vi "Dashboard Main.vi"() -> ()   [LabVIEW 2012]
uses:
  <vilib>/event_ctls.llb/eventvkey.ctl
  <vilib>/Utility/config.llb/Read Key (String).vi
  <vilib>/Utility/config.llb/Read Key (I32).vi
  <vilib>/Utility/config.llb/Write Key (String).vi
  <vilib>/Utility/config.llb/Write Key (I32).vi
  <vilib>/Utility/config.llb/NI_LVConfig.lvlib
panel:
  out "Mode":T1(ring)=enum."Auto Disabled"
  in  "Viewer":enum32{"Camera Image", "Variables"}(tab)
  out "Mbps":dbl format="%#.1g"
  in  "Enable":bool=TRUE
  in  "DB Camera Config":bool
  out "Mbps":bool
  out "fps":dbl format="%#.1g"
  out "Image Error Message":string="Timeout in Camera Communications"
  out "Camera Image":T2(plugin-control)
  out "Camera Image 2":T2(plugin-control)
  in  "Camera Settings":T3={"Frame Rate"=15, "Compression"=30, "Size"=1} {"Frame Rate" scale=1.0..30.0; "Size" items=["640x480", "320x240", "160x120"]}
  out "Camera IP 2":string
  out "Camera IP":string
  out "fps 2":dbl format="%#.1g"
  out "Mbps 2":dbl format="%#.1g"
  in  "Enable 2":bool=TRUE
  in  "FR":i32=15
  out "Tree":string(tree)
  in  "Dashboard Tab":enum32{"Operation", "Test", "Checklist"}(tab)
  in  "Auton Selector":T4(radio)
  in  "Auton Refresh":bool
  out "AutonFiles":string[](array[string])
  in  "Slider":dbl(slide) scale=0.0..100.0 scale format="%#_3g"
  in  "On/Off":bool caption="Solenoid"
  in  "Test Name":u16(ring) items=["Select the test to run...", "Example Test", "-------------------------------", "List of tests is built in robot code.", "Replace with your own automated tests."]
  in  "Test Tree":string(tree)
  in  "Motor":cluster{"Value":dbl, "Enable":bool} {"Value" scale=-1.0..1.0 scale format="%#_3g"}
  out "Progress":T5 {"Test Progress" scale=0.0..100.0}
  in  "Rev/Fwd":cluster{"Forward":bool, "Reverse":bool}
  in  "Ring":u16(ring) items=["Auto", "Fixed indoor", "Fixed outdoor 1", "Fixed outdoor 2", "Fixed fluorescent 1", "Fixed fluorescent 2", "Hold current"]
  in  "Listbox":i32(listbox)
  out "Robot IP":string
  out "Battery Value":dbl(slide) scale=0.0..14.0 scale format="%#_2e"
  out "Battery":sgl(graph)
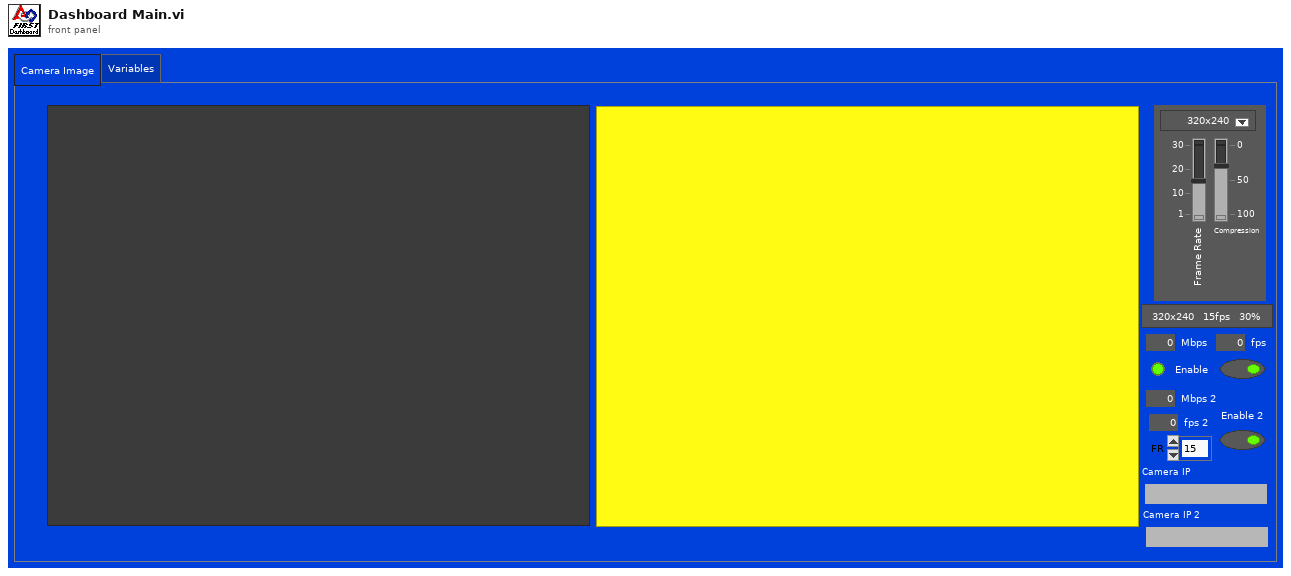
[diagram p1: front panel]
types:
  T1 = enum8{"Tele-Op Disabled", "Tele-Op Enabled", "Auto Disabled", "Auto Enabled", "Test Disabled", "Test Enabled", ""}
  T2 = typedef "IMAQ Image.ctl" = refnum<image>
  T3 = cluster{"Frame Rate":i32, "Compression":i32, "Size":u16}
  T4 = enum32{"Boolean 1", "Boolean 2", "Boolean 3", "Boolean 4", "Boolean 5", "Boolean 6", "Boolean 7", "Boolean 8"}
  T5 = cluster{"Test Progress":u8, "Test Progress Text":string}
  T6 = typedef "Image Type" = u32
  T7 = cluster{"Competition mode":bool, "Robot Link":bool, "Autonomous":bool, "Enabled":bool, "E-Stop":bool, "Simulated":bool, "TestMode":bool, "Docked Window":bool}
  T8 = typedef "LVRectTypeDef.ctl" = cluster{"Left":i16, "Top":i16, "Right":i16, "Bottom":i16}
  T9 = typedef "NI_LVConfig.lvlib/Config Data RefNum.ctl" = refnum<k1>
  T10 = typedef "eventvkey.ctl" = enum16{"ASCII", "Enter", "Return", "Shift", "Ctrl", "Alt", "Cmd", "Opt", "Caps", "NumLock", "Clear", "Break", "Up", "Down", "Left", "Right", "Insert", "Delete", "Home", "End", "PageUp", "PageDown", "Escape", "Help", "Pause", "ScrollLock", "F1", "F2", "F3", "F4", "F5", "F6", "F7", "F8", "F9", "F10", "F11", "F12", "F13", "F14", "F15", "F16", "F17", "F18", "F19", "F20", "F21", "F22", "F23", "F24", "Play", "VolumeUp", "VolumeDown", "Mute", "Two Byte Char"}
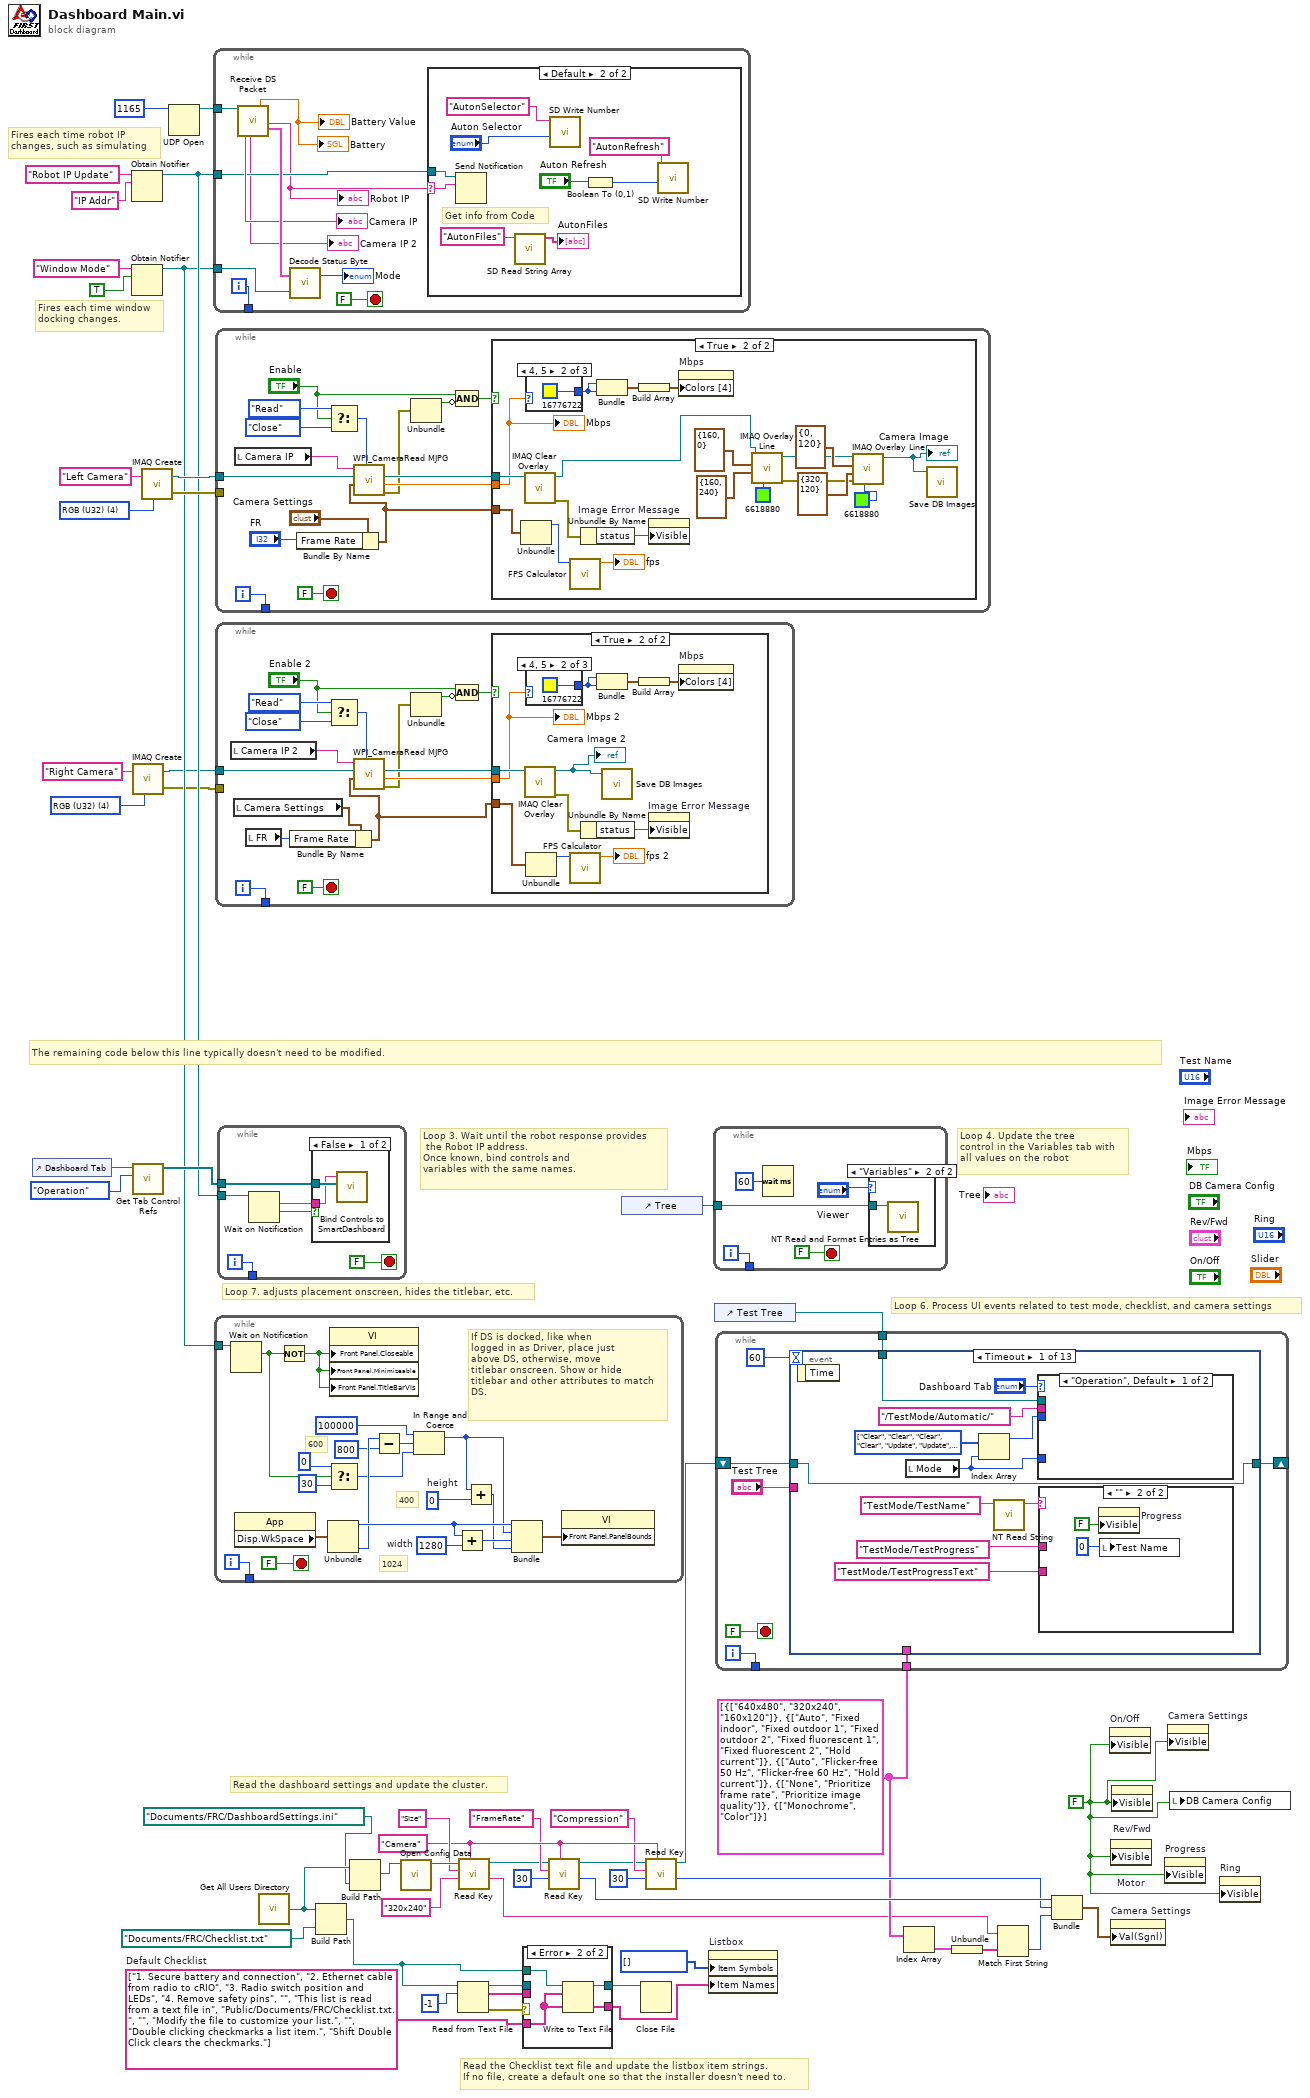
[diagram p0: block diagram]
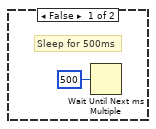
[diagram p2: hidden frame]
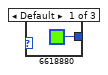
[diagram p3: hidden frame]
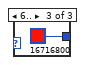
[diagram p4: hidden frame]
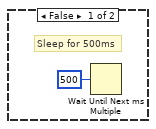
[diagram p6: hidden frame]
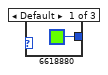
[diagram p7: hidden frame]
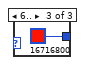
[diagram p8: hidden frame]
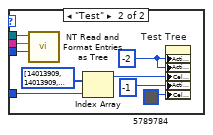
[diagram p10: hidden frame]
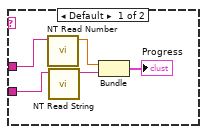
[diagram p11: hidden frame]
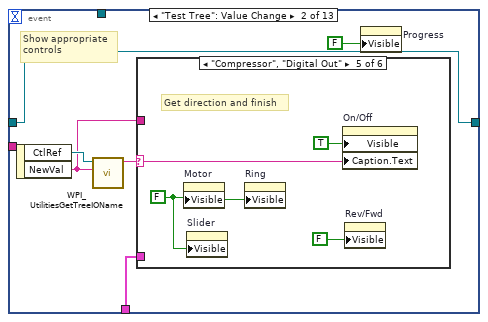
[diagram p12: hidden frame]
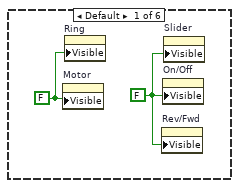
[diagram p13: hidden frame]
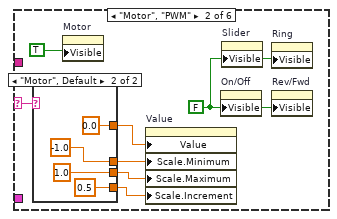
[diagram p14: hidden frame]
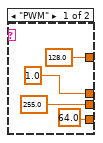
[diagram p15: hidden frame]
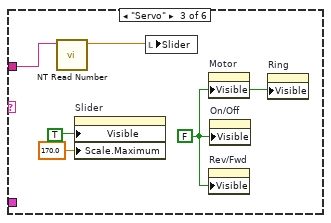
[diagram p16: hidden frame]
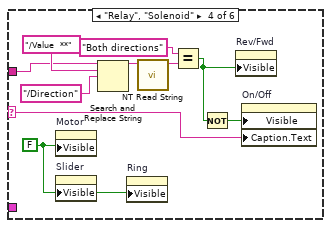
[diagram p17: hidden frame]
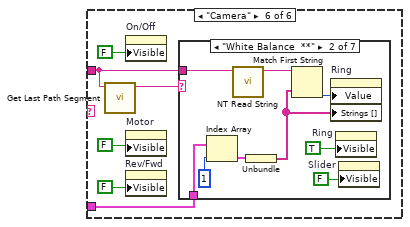
[diagram p18: hidden frame]
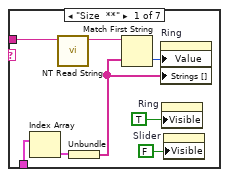
[diagram p19: hidden frame]
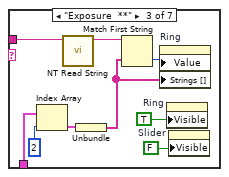
[diagram p20: hidden frame]
diagram:
  w3 = T6 4 items=["Grayscale (U8)", "Grayscale (I16)", "Grayscale (SGL)", "Complex (CSG)", "RGB (U32)", "HSL (U32)", "RGB (U64)"] ("Image Type")
  w25 = "Camera"
  w17 = cluster{string[]}[] [{["640x480", "320x240", "160x120"]}, {["Auto", "Fixed indoor", "Fixed outdoor 1", "Fixed outdoor 2", "Fixed fluorescent 1", "Fixed fluorescent 2", "Hold current"]}, {["Auto", "Flicker-free 50 Hz", "Flicker-free 60 Hz", "Hold current"]}, {["None", "Prioritize frame rate", "Prioritize image quality"]}, {["Monochrome", "Color"]}]
  w33 = string[] ["1. Secure battery and connection", "2. Ethernet cable from radio to cRIO", "3. Radio switch position and LEDs", "4. Remove safety pins", "", "This list is read from a text file in", "Public/Documents/FRC/Checklist.txt.", "", "Modify the file to customize your list.", "", "Double clicking checkmarks a list item.", "Shift Double Click clears the checkmarks."]  # Default Checklist
  w31 = FALSE ("Visible")
  w52 = T6 4 items=["Grayscale (U8)", "Grayscale (I16)", "Grayscale (SGL)", "Complex (CSG)", "RGB (U32)", "HSL (U32)", "RGB (U64)"] ("Image Type")
  # "Fires each time robot IP\nchanges, such as simulating"
  # "Fires each time window\ndocking changes."
  # "Read the Checklist text file and update the listbox item strings.\nIf no file, create a default one so that the installer doesn't need to."
  # "The remaining code below this line typically doesn't need to be modified."
  # "Loop 6. Process UI events related to test mode, checklist, and camera settings"
  # "Read the dashboard settings and update the cluster."
  # "Loop 4. Update the tree\ncontrol in the Variables tab with\nall values on the robot"
  # "Loop 3. Wait until the robot response provides\n the Robot IP address.\nOnce known, bind controls and\nvariables with the same names."
  # "Loop 7. adjusts placement onscreen, hides the titlebar, etc."
  n1 = control-ref of="Dashboard Tab"() -> (w47:refnum<vi>)
  n2 = Obtain Notifier(name (unnamed)="Robot IP Update", notification data type="IP Addr" ("name (unnamed)")) -> (notifier out=w44:refnum<notifier>)  [unwired: 2 in, 2 out]
  n3 = Obtain Notifier(name (unnamed)="Window Mode", notification data type=TRUE) -> (notifier out=w37:refnum<notifier>)  [unwired: 2 in, 2 out]
  n4 = call "IMAQ Create"("Image Name"="Right Camera", "Image Type"=w3) -> ("New Image"=w2:T2, "error out"=w1:errorcluster)  [unwired: 2 in, 1 out]
  n5 = call <vilib>:"Get Tab Control Refs.vi"("Page Index"=enum32{"Operation", "Test"}."Operation" ("Dashboard Tab"), "TabControl in"=w47) -> ("ControlsOnPage"=w48:refnum<vi>[])  [unwired: 9 in]
  n6 = call "IMAQ Create"("Image Name"="Left Camera", "Image Type"=w52) -> ("New Image"=w50:T2, "error out"=w49:errorcluster)  [unwired: 2 in, 1 out]
  n7 = UDP Open(11:u16 1165 ("port")) -> (port=w53:refnum<k16>)  [unwired: 2 in, 4 out]
  n8 = while {
    tunnel: w53 -> [w63]
    tunnel: w44 -> [w57]
    tunnel: w37 -> [w61]
    tunnel: [w58] -> _
    i -> [w58]
    stop <- FALSE stop-if-true
    n9 = call "Receive DS Packet.vi"("Recv Socket"=w63) -> ("Camera IP Address"=→"Camera IP":string, "Camera IP Address 2"=→"Camera IP 2":string, "Battery"=→"Battery" →"Battery Value":sgl, "Robot IP Address"=w56:string, "Status"=w64:T7)  [unwired: 8 in, 6 out]
    "Robot IP" <- w56
    n10 = call "Decode Status Byte.vi"("Window Mode Notifier"=w61, "Status"=w64) -> ("Mode"=→"Mode":T1)  [unwired: 1 out]
    n11 = case shown="Default" w56 {
      selector: w56 -> [_ w73]
      tunnel: w57 -> [_ w74]
      frame "0.0.0.0" {
        # "Robot not responding, don't poll the variables"
      }
      frame Default {
        # "Get info from Code"
        n12 = Send Notification(notification=w73, notifier=w74) -> ()  [unwired: 1 in, 2 out]
        n13 = call <vilib>:"SD Read String Array.vi"("Name"="AutonFiles") -> ("String Array"=→"AutonFiles":string[])  [unwired: 9 in, 1 out]
        n14 = call <vilib>:"SD Write Number.vi"("Numeric"="Auton Selector", "Name"="AutonSelector") -> ()  [unwired: 8 in, 2 out]
        n15 = Boolean To (0,1)(Boolean="Auton Refresh") -> (0, 1=w67:i16)
        n16 = call <vilib>:"SD Write Number.vi"("Numeric"=w67, "Name"="AutonRefresh") -> ()  [unwired: 8 in, 2 out]
      }
    }
  }
  n17 = while {
    tunnel: w37 -> [w93]
    tunnel: [w91] -> _
    i -> [w91]
    stop <- FALSE stop-if-true
    w83 = 1280  # width
    w86 = 0  # height
    # "600"
    # "1024"
    # "400"
    # "If DS is docked, like when\nlogged in as Driver, place just\nabove DS, otherwise, move\ntitlebar onscreen. Show or hide\ntitlebar and other attributes to match\nDS."
    n18 = Wait on Notification(notifier=w93) -> (notification=w78:bool)  [unwired: 3 in, 3 out]
    n19 = property class="App"() -> ("Disp.WkSpace"=w89:T8)  [unwired: 2 in, 2 out]
    n20 = Not(x=w78) -> (.not. x?=w92:bool)
    n21 = Unbundle(w89) -> ("Left"=w87:i16, "Bottom"=w84:i16)  [unwired: 2 out]
    n22 = Select(t=0, s=w78, f=30) -> (s? t:f=w77:i32)
    n23 = property class="VI"("Front Panel.Closeable"=w92, "Front Panel.Minimizeable"=w92, "Front Panel.TitleBarVis"=w92) -> ()  [unwired: 2 in, 2 out]
    n24 = Subtract(x=w84, y=800) -> (x-y=w81:i32)
    n25 = In Range and Coerce(upper limit=100000, x=w81, lower limit=w77) -> (coerced(x)=w75:i32)  [unwired: 1 out]
    n26 = Add(x=w87, y=w83) -> (x+y=w88:i32)
    n27 = Add(x=w75, y=w86) -> (x+y=w85:i32)
    n28 = Bundle("Left"=w87, w75, w88, w85) -> (w90:cluster{"Left":i16, i32, i32, i32})  [unwired: 1 out]
    n29 = property class="VI"("Front Panel.PanelBounds"=w90) -> ()  [unwired: 2 in, 2 out]
  }
  n30 = while {
    tunnel: w50 -> [w107]
    tunnel: w49 -> [_]
    tunnel: [w109] -> _
    i -> [w109]
    stop <- FALSE stop-if-true
    n31 = local read "Camera IP"() -> (w108:string)
    n32 = Bundle By Name(cluster="Camera Settings", "Frame Rate"="FR") -> (w95:T3)
    n33 = Select(t=enum16{"Read", "Reopen", "Close"}."Read" ("Operation"), s="Enable", f=enum16{"Read", "Reopen", "Close"}."Close" ("Operation")) -> (s? t:f=w102:enum16{"Read", "Reopen", "Close"})
    n34 = call <vilib>:"WPI_CameraRead MJPG.vi"("Operation"=w102, "Camera Settings"=w95, "Image"=w107, "address"=w108) -> ("error out"=w101:errorcluster, "Bandwidth (kbps)"=w105:dbl, "Image Out"=w106:T2)  [unwired: 5 in]
    n35 = Unbundle(w101) -> ("status"=w99:bool)  [unwired: 2 out]
    n36 = Compound Arithmetic op=AND("Enable", invert w99) -> (w98:bool)
    n37 = case shown="True" w98 {
      tunnel: w95 -> [_ w123]
      tunnel: w106 -> [_ w126]
      tunnel: w105 -> [_ w125]
      frame False {
        # "Sleep for 500ms"
        n38 = Wait Until Next ms Multiple(millisecond multiple=u32 500) -> ()  [unwired: 1 out]
      }
      frame True {
        n39 = Unbundle(w123) -> ("Frame Rate"=w113:i32)  [unwired: 2 out]
        n40 = call "IMAQ Clear Overlay"("Image"=w126) -> ("error out"=w130:errorcluster, "Image Out"=w115:T2)  [unwired: 2 in, 7 out]
        n41 = case shown="4, 5" w125 {
          tunnel: [u32 6618880 ("Color Box") u32 16776722 ("Color Box") u32 16716800 ("Color Box")] -> w127
          frame Default {
          }
          frame 4, 5 {
          }
          frame 6.. {
          }
        }
        n42 = call "FPS Calculator.vi"("Average Count"=w113) -> ("fps"=→"fps":dbl)  [unwired: 10 in]
        n43 = Unbundle By Name(w130) -> ("status"=w131:bool)
        n44 = Bundle("Color Box"=w127, "Color Box"=w127) -> (w129:cluster{"Color Box":u32, "Color Box":u32})  [unwired: 1 out]
        n45 = Build Array(w129) -> (w128:cluster{"Color Box":u32, "Color Box":u32}[])
        n46 = property on="Image Error Message" class="Str"("Visible"=w131) -> ()  [unwired: 2 in, 2 out]
        n47 = property on="Mbps" class="Bool (strict)"("Colors [4]"=w128) -> ()  [unwired: 2 in, 2 out]
        n48 = call "IMAQ Overlay Line"("Color"=u32 6618880, "End Point"=cluster{"X":i32, "Y":i32} {"X"=160, "Y"=240}, "Start Point"=cluster{"X":i32, "Y":i32} {"X"=160, "Y"=0}, "Image"=w115) -> ("error out"=w120:errorcluster, "Image Out"=w119:T2)  [unwired: 6 in]
        n49 = call "IMAQ Overlay Line"("Color"=u32 6618880, "error in (no error)"=w120, "End Point"=cluster{"X":i32, "Y":i32} {"X"=320, "Y"=120}, "Start Point"=cluster{"X":i32, "Y":i32} {"X"=0, "Y"=120}, "Image"=w119) -> ("Image Out"=w114:T2)  [unwired: 5 in, 1 out]
        "Camera Image" <- w114
        n50 = call "Save DB Images.vi"("Image"=w114) -> ()  [unwired: 2 in, 1 out]
        "Mbps" <- w125
      }
    }
  }
  n51 = while {
    tunnel: w2 -> [w147]
    tunnel: [w149] -> _
    tunnel: w1 -> [_]
    i -> [w149]
    stop <- FALSE stop-if-true
    n52 = local read "Camera IP 2"() -> (w148:string)
    n53 = local read "Camera Settings"() -> (w136:T3)
    n54 = local read "FR"() -> (w137:i32)
    n55 = Bundle By Name(cluster=w136, "Frame Rate"=w137) -> (w135:T3)
    n56 = Select(t=enum16{"Read", "Reopen", "Close"}."Read" ("Operation"), s="Enable 2", f=enum16{"Read", "Reopen", "Close"}."Close" ("Operation")) -> (s? t:f=w142:enum16{"Read", "Reopen", "Close"})
    n57 = call <vilib>:"WPI_CameraRead MJPG.vi"("Operation"=w142, "Camera Settings"=w135, "Image"=w147, "address"=w148) -> ("error out"=w141:errorcluster, "Bandwidth (kbps)"=w145:dbl, "Image Out"=w146:T2)  [unwired: 5 in]
    n58 = Unbundle(w141) -> ("status"=w139:bool)  [unwired: 2 out]
    n59 = Compound Arithmetic op=AND("Enable 2", invert w139) -> (w138:bool)
    n60 = case shown="True" w138 {
      tunnel: w135 -> [_ w154]
      tunnel: w146 -> [_ w157]
      tunnel: w145 -> [_ w156]
      frame False {
        # "Sleep for 500ms"
        n61 = Wait Until Next ms Multiple(millisecond multiple=u32 500) -> ()  [unwired: 1 out]
      }
      frame True {
        n62 = call "IMAQ Clear Overlay"("Image"=w157) -> ("error out"=w161:errorcluster, "Image Out"=w152:T2)  [unwired: 2 in, 7 out]
        "Camera Image 2" <- w152
        n63 = case shown="4, 5" w156 {
          tunnel: [u32 6618880 ("Color Box") u32 16776722 ("Color Box") u32 16716800 ("Color Box")] -> w158
          frame Default {
          }
          frame 4, 5 {
          }
          frame 6.. {
          }
        }
        n64 = Unbundle(w154) -> ("Frame Rate"=w153:i32)  [unwired: 2 out]
        n65 = call "FPS Calculator.vi"("Average Count"=w153) -> ("fps"=→"fps 2":dbl)  [unwired: 10 in]
        n66 = Unbundle By Name(w161) -> ("status"=w162:bool)
        n67 = Bundle("Color Box"=w158, "Color Box"=w158) -> (w160:cluster{"Color Box":u32, "Color Box":u32})  [unwired: 1 out]
        n68 = call "Save DB Images.vi"("Image"=w152) -> ()  [unwired: 2 in, 1 out]
        n69 = Build Array(w160) -> (w159:cluster{"Color Box":u32, "Color Box":u32}[])
        n70 = property on="Image Error Message" class="Str"("Visible"=w162) -> ()  [unwired: 2 in, 2 out]
        n71 = property on="Mbps" class="Bool (strict)"("Colors [4]"=w159) -> ()  [unwired: 2 in, 2 out]
        "Mbps 2" <- w156
      }
    }
  }
  n72 = while {
    tunnel: w48 -> [w171]
    tunnel: w44 -> [w168]
    tunnel: [w166] -> _
    i -> [w166]
    stop <- FALSE stop-if-true
    n73 = Wait on Notification(notifier=w168) -> (notification=w167:string, timed out?=w169:bool)  [unwired: 3 in, 2 out]
    n74 = case shown="False" w169 {
      tunnel: w171 -> [w173 _]
      tunnel: w167 -> [w172 _]
      frame False {
        n75 = call <vilib>:"Bind Controls to SmartDashboard.vi"("Bound Control Refs"=w173, "Server IP Address"=w172) -> ()  [unwired: 10 in]
      }
      frame True {
      }
    }
  }
  n76 = call "Get All Users Directory.vi"() -> ("All User Path"=w30:path)
  n77 = Build Path(base path=w30, name or relative path=path "Documents/FRC/Checklist.txt") -> (appended path=w34:path)
  n78 = Build Path(base path=w30, name or relative path=path "Documents/FRC/DashboardSettings.ini") -> (appended path=w29:path)
  n79 = call <vilib>:"Open Config Data.vi"("configuration file path"=w29) -> ("refnum"=w28:T9)  [unwired: 8 in, 2 out]
  n80 = Read from Text File(file (use dialog)=w34, count=-1 ("timeout ms (25000)")) -> (refnum out=w12:refnum<file>, text=w35:string[], error out=w36:errorcluster)  [unwired: 2 in, 1 out]
  n81 = call-poly <vilib>:"Read Key.vi"("section"=w25, "default value"="320x240", "key"="Size", "refnum"=w28) -> ("value"=w15:string, "refnum out"=w10:T9)  [unwired: 2 in, 4 out]
  n82 = case shown="Error" w36 {
    tunnel: w35 -> [w175 _]
    tunnel: [w175 w177] -> w32
    tunnel: w33 -> [_ w177]
    tunnel: w34 -> [_ w178]
    tunnel: [w174 w176] -> w11
    tunnel: w12 -> [w174 _]
    frame No Error {
    }
    frame Error {
      n83 = Write to Text File(file (use dialog)=w178, text=w177) -> (refnum out=w176:refnum<file>)  [unwired: 2 in, 2 out]
    }
  }
  n84 = call-poly <vilib>:"Read Key.vi"("section"=w25, "default value"=30, "key"="FrameRate", "refnum"=w10) -> ("value"=w20:i32, "refnum out"=w9:T9)  [unwired: 1 in, 5 out]
  n85 = control-ref of="Tree"() -> (w6:refnum<vi>)
  n86 = Close File(refnum=w11) -> ()  [unwired: 1 in, 2 out]
  n87 = call-poly <vilib>:"Read Key.vi"("section"=w25, "default value"=30, "key"="Compression", "refnum"=w9) -> ("value"=w19:i32, "refnum out"=w7:T9)  [unwired: 1 in, 5 out]
  n88 = property on="Listbox" class="LstBox (strict)"("Item Symbols"=i32[] [], "Item Names"=w32) -> ()  [unwired: 2 in, 2 out]
  n89 = while {
    tunnel: [w180] -> _
    tunnel: w6 -> [w179]
    i -> [w180]
    stop <- FALSE stop-if-true
    n90 = Wait (ms)(milliseconds to wait=u32 60) -> ()  [unwired: 1 out]
    n91 = case shown="\"Variables\"" "Viewer" {
      tunnel: w179 -> [_ w184]
      frame Default {
      }
      frame "Variables" {
        n92 = call <vilib>:"NT Read and Format Entries as Tree.vi"("Tree Refnum"=w184) -> ()  [unwired: 9 in, 2 out]
      }
    }
  }
  n93 = control-ref of="Test Tree"() -> (w5:refnum<vi>)
  n94 = while {
    tunnel: w17 -> [w189]
    shift-right: [w188] -> _
    shift-left: w7 -> [w187]
    tunnel: [w186] -> _
    tunnel: w5 -> [w185]
    i -> [w186]
    stop <- FALSE stop-if-true
    n95 = event shown="[0] Timeout" {
      selector: _ -> [_ _ _ _ _ _ _ _ _ _ _ _ _]
      dyn-events: _ -> [_ _ _ _ _ _ _ _ _ _ _ _ _]
      timeout: u32 60 ("milliseconds to wait") -> [_ _ _ _ _ _ _ _ _ _ _ _ _]
      tunnel: w185 -> [w199 _ _ _ _ _ _ _ _ _ _ _ _]
      tunnel: "Test Tree" -> [_ _ _ _ _ _ _ _ w393 w401 w403 w407 w415]
      tunnel: w189 -> [_ w221 _ _ _ _ w357 w387 _ _ _ _ _]
      tunnel: [w193 w220 _ w323 w331 w343 w356 w380 w392 w399 w402 w406 w414] -> w188
      tunnel: w187 -> [w193 w220 _ w323 w331 w343 w355 w380 w392 w399 w402 w406 w414]
      event Timeout {
        w198 = enum16{"Update", "Clear"}[] [enum."Clear", enum."Clear", enum."Clear", enum."Clear", enum."Update", enum."Update", enum."Clear"] items=["Update", "Clear"]
        n96 = event-data() -> ()  [unwired: 1 in, 1 out]
        n97 = local read "Mode"() -> (w196:T1)
        n98 = Index Array(array=w198, index=w196) -> (element=w197:enum16{"Update", "Clear"})
        n99 = call <vilib>:"NT Read String.vi"("Name"="TestMode/TestName") -> ("String"=w202:string)  [unwired: 9 in, 1 out]
        n100 = case shown="\"Operation\", Default" "Dashboard Tab" {
          tunnel: w199 -> [_ w212]
          tunnel: "/TestMode/Automatic/" ("Name Pattern") -> [_ w211]
          tunnel: w197 -> [_ w210]
          tunnel: w196 -> [_ w208]
          frame "Operation", Default {
          }
          frame "Test" {
            w207 = -2 ("Active Item:Row Number")
            n101 = call <vilib>:"NT Read and Format Entries as Tree.vi"("Operation"=w210, "Name Pattern"=w211, "Tree Refnum"=w212) -> ()  [unwired: 7 in, 2 out]
            n102 = Index Array(array=u32[] [14013909, 14013909, 14013909, 14013909, 14013909, 16777215, 14013909], index=w208) -> (element=w206:u32)
            n103 = property on="Test Tree" class="Tree (strict)"("Active Item Row Number"=w207, "ActiveColNum"=w207, "CellBG"=w206, "Active Item Row Number"=-1 ("Active Item:Row Number"), "CellBG"=u32 5789784 ("Color Box")) -> ()  [unwired: 2 in, 2 out]
          }
        }
        n104 = case shown="\"\"" w202 {
          tunnel: "TestMode/TestProgress" ("Name") -> [w214 _]
          tunnel: "TestMode/TestProgressText" ("Name") -> [w213 _]
          frame Default {
            n105 = call <vilib>:"NT Read Number.vi"("Name"=w214) -> ("Numeric"=w215:dbl)  [unwired: 9 in, 1 out]
            n106 = call <vilib>:"NT Read String.vi"("Name"=w213) -> ("String"=w216:string)  [unwired: 9 in, 1 out]
            n107 = Bundle("Numeric"=w215, "String"=w216) -> (→"Progress":cluster{"Numeric":dbl, "String":string})  [unwired: 1 in]
          }
          frame "" {
            n108 = property on="Progress" class="Clust (strict)"("Visible"=FALSE) -> ()  [unwired: 2 in, 2 out]
            n109 = local write "Test Name"(u16 0) -> ()
          }
        }
      }
      event "Test Tree": Value Change {
        # "Show appropriate\ncontrols"
        n110 = event-data() -> ("CtlRef"=w224:refnum<vi>, "NewVal"=w222:string)  [unwired: 1 in]
        n111 = call <vilib>:"WPI_UtilitiesGetTreeIOName.vi"("NewVal"=w222, "TreeControl in"=w224) -> ("I/O Name"=w225:string)  [unwired: 9 in]
        n112 = case shown="\"Compressor\", \"Digital Out\"" w225 {
          selector: w225 -> [_ w232 _ w250 w259 _]
          tunnel: w222 -> [_ _ w247 w249 _ w266]
          tunnel: w221 -> [_ _ _ _ _ w265]
          frame Default {
            w227 = FALSE ("Visible")
            w226 = FALSE ("Visible")
            n113 = property on="Motor" class="Clust (strict)"("Visible"=w226) -> ()  [unwired: 2 in, 2 out]
            n114 = property on="Ring" class="Ring (strict)"("Visible"=w226) -> ()  [unwired: 2 in, 2 out]
            n115 = property on="Rev/Fwd" class="Clust (strict)"("Visible"=w227) -> ()  [unwired: 2 in, 2 out]
            n116 = property on="On/Off" class="Bool (strict)"("Visible"=w227) -> ()  [unwired: 2 in, 2 out]
            n117 = property on="Slider" class="Slide (strict)"("Visible"=w227) -> ()  [unwired: 2 in, 2 out]
          }
          frame "Motor", "PWM" {
            w233 = FALSE ("Visible")
            n118 = case shown="\"Motor\", Default" w232 {
              tunnel: [1.0 ("Value") -1.0 ("Value")] -> w231
              tunnel: [255.0 ("Value") 1.0 ("Value")] -> w230
              tunnel: [128.0 ("Value") 0.0 ("Value")] -> w229
              tunnel: [64.0 ("Value") 0.5 ("Value")] -> w228
              frame "PWM" {
              }
              frame "Motor", Default {
              }
            }
            n119 = property on="Motor" class="Clust (strict)"("Visible"=TRUE) -> ()  [unwired: 2 in, 2 out]
            n120 = property on="Value" class="Slide (strict)"("Value"=w229, "Scale.Minimum"=w231, "Scale.Maximum"=w230, "Scale.Increment"=w228) -> ()  [unwired: 2 in, 2 out]
            n121 = property on="On/Off" class="Bool (strict)"("Visible"=w233) -> ()  [unwired: 2 in, 2 out]
            n122 = property on="Slider" class="Slide (strict)"("Visible"=w233) -> ()  [unwired: 2 in, 2 out]
            n123 = property on="Ring" class="Ring (strict)"("Visible"=w233) -> ()  [unwired: 2 in, 2 out]
            n124 = property on="Rev/Fwd" class="Clust (strict)"("Visible"=w233) -> ()  [unwired: 2 in, 2 out]
          }
          frame "Servo" {
            w245 = FALSE ("Visible")
            n125 = call <vilib>:"NT Read Number.vi"("Name"=w247) -> ("Numeric"=w246:dbl)  [unwired: 9 in, 1 out]
            n126 = property on="Slider" class="Slide (strict)"("Visible"=TRUE, "Scale.Maximum"=170.0 ("Scale.Range:Maximum")) -> ()  [unwired: 2 in, 2 out]
            n127 = local write "Slider"(w246) -> ()
            n128 = property on="Motor" class="Clust (strict)"("Visible"=w245) -> ()  [unwired: 2 in, 2 out]
            n129 = property on="Rev/Fwd" class="Clust (strict)"("Visible"=w245) -> ()  [unwired: 2 in, 2 out]
            n130 = property on="On/Off" class="Bool (strict)"("Visible"=w245) -> ()  [unwired: 2 in, 2 out]
            n131 = property on="Ring" class="Ring (strict)"("Visible"=w245) -> ()  [unwired: 2 in, 2 out]
          }
          frame "Relay", "Solenoid" {
            w248 = FALSE ("Visible")
            n132 = property on="Motor" class="Clust (strict)"("Visible"=w248) -> ()  [unwired: 2 in, 2 out]
            n133 = property on="Slider" class="Slide (strict)"("Visible"=w248) -> ()  [unwired: 2 in, 2 out]
            n134 = Search and Replace String(input string=w249, search string="/Value  **", replace string="/Direction") -> (result string=w255:string)  [unwired: 5 in, 3 out]
            n135 = property on="Ring" class="Ring (strict)"("Visible"=w248) -> ()  [unwired: 2 in, 2 out]
            n136 = call <vilib>:"NT Read String.vi"("Name"=w255) -> ("String"=w253:string)  [unwired: 9 in, 1 out]
            n137 = Equal?(x="Both directions", y=w253) -> (x = y?=w251:bool)
            n138 = Not(x=w251) -> (.not. x?=w252:bool)
            n139 = property on="Rev/Fwd" class="Clust (strict)"("Visible"=w251) -> ()  [unwired: 2 in, 2 out]
            n140 = property on="On/Off" class="Bool (strict)"("Visible"=w252, "Caption.Text"=w250) -> ()  [unwired: 2 in, 2 out]
          }
          frame "Compressor", "Digital Out" {
            w258 = FALSE ("Visible")
            # "Get direction and finish"
            n141 = property on="Motor" class="Clust (strict)"("Visible"=w258) -> ()  [unwired: 2 in, 2 out]
            n142 = property on="Slider" class="Slide (strict)"("Visible"=w258) -> ()  [unwired: 2 in, 2 out]
            n143 = property on="Ring" class="Ring (strict)"("Visible"=w258) -> ()  [unwired: 2 in, 2 out]
            n144 = property on="On/Off" class="Bool (strict)"("Visible"=TRUE, "Caption.Text"=w259) -> ()  [unwired: 2 in, 2 out]
            n145 = property on="Rev/Fwd" class="Clust (strict)"("Visible"=FALSE) -> ()  [unwired: 2 in, 2 out]
          }
          frame "Camera" {
            n146 = call <vilib>:"Get Last Path Segment.vi"("String in"=w266) -> ("String out"=w267:string)  [unwired: 10 in]
            n147 = property on="On/Off" class="Bool (strict)"("Visible"=FALSE) -> ()  [unwired: 2 in, 2 out]
            n148 = property on="Motor" class="Clust (strict)"("Visible"=FALSE) -> ()  [unwired: 2 in, 2 out]
            n149 = property on="Rev/Fwd" class="Clust (strict)"("Visible"=FALSE) -> ()  [unwired: 2 in, 2 out]
            n150 = case shown="\"White Balance  **\"" w267 {
              tunnel: w266 -> [w273 w282 w291 w300 w309 _ w315]
              tunnel: w265 -> [w271 w279 w288 w297 w306 _ _]
              frame "Size  **" {
                n151 = Index Array(array=w271) -> (element=w270:cluster{string[]})  [unwired: 1 in]
                n152 = call <vilib>:"NT Read String.vi"("Name"=w273) -> ("String"=w272:string)  [unwired: 9 in, 1 out]
                n153 = Unbundle(w270) -> (w268:string[])
                n154 = Match First String(2:w268, 3:w272) -> (0:w269:i32)  [unwired: 1 out]
                n155 = property on="Ring" class="Ring (strict)"("Value"=w269, "Strings []"=w268) -> ()  [unwired: 2 in, 2 out]
                n156 = property on="Ring" class="Ring (strict)"("Visible"=TRUE) -> ()  [unwired: 2 in, 2 out]
                n157 = property on="Slider" class="Slide (strict)"("Visible"=FALSE) -> ()  [unwired: 2 in, 2 out]
              }
              frame "White Balance  **" {
                n158 = Index Array(array=w279, index=1) -> (element=w280:cluster{string[]})
                n159 = call <vilib>:"NT Read String.vi"("Name"=w282) -> ("String"=w281:string)  [unwired: 9 in, 1 out]
                n160 = Unbundle(w280) -> (w277:string[])
                n161 = Match First String(2:w277, 3:w281) -> (0:w276:i32)  [unwired: 1 out]
                n162 = property on="Ring" class="Ring (strict)"("Value"=w276, "Strings []"=w277) -> ()  [unwired: 2 in, 2 out]
                n163 = property on="Ring" class="Ring (strict)"("Visible"=TRUE) -> ()  [unwired: 2 in, 2 out]
                n164 = property on="Slider" class="Slide (strict)"("Visible"=FALSE) -> ()  [unwired: 2 in, 2 out]
              }
              frame "Exposure  **" {
                n165 = Index Array(array=w288, index=2) -> (element=w289:cluster{string[]})
                n166 = call <vilib>:"NT Read String.vi"("Name"=w291) -> ("String"=w290:string)  [unwired: 9 in, 1 out]
                n167 = Unbundle(w289) -> (w285:string[])
                n168 = Match First String(2:w285, 3:w290) -> (0:w286:i32)  [unwired: 1 out]
                n169 = property on="Ring" class="Ring (strict)"("Value"=w286, "Strings []"=w285) -> ()  [unwired: 2 in, 2 out]
                n170 = property on="Ring" class="Ring (strict)"("Visible"=TRUE) -> ()  [unwired: 2 in, 2 out]
                n171 = property on="Slider" class="Slide (strict)"("Visible"=FALSE) -> ()  [unwired: 2 in, 2 out]
              }
              frame "Exposure Priority  **" {
                n172 = Index Array(array=w297, index=3) -> (element=w298:cluster{string[]})
                n173 = call <vilib>:"NT Read String.vi"("Name"=w300) -> ("String"=w299:string)  [unwired: 9 in, 1 out]
                n174 = Unbundle(w298) -> (w294:string[])
                n175 = Match First String(2:w294, 3:w299) -> (0:w295:i32)  [unwired: 1 out]
                n176 = property on="Ring" class="Ring (strict)"("Value"=w295, "Strings []"=w294) -> ()  [unwired: 2 in, 2 out]
                n177 = property on="Ring" class="Ring (strict)"("Visible"=TRUE) -> ()  [unwired: 2 in, 2 out]
                n178 = property on="Slider" class="Slide (strict)"("Visible"=FALSE) -> ()  [unwired: 2 in, 2 out]
              }
              frame "Color Enable  **" {
                n179 = Index Array(array=w306, index=4) -> (element=w307:cluster{string[]})
                n180 = call <vilib>:"NT Read String.vi"("Name"=w309) -> ("String"=w308:string)  [unwired: 9 in, 1 out]
                n181 = Unbundle(w307) -> (w303:string[])
                n182 = Match First String(2:w303, 3:w308) -> (0:w304:i32)  [unwired: 1 out]
                n183 = property on="Ring" class="Ring (strict)"("Value"=w304, "Strings []"=w303) -> ()  [unwired: 2 in, 2 out]
                n184 = property on="Ring" class="Ring (strict)"("Visible"=TRUE) -> ()  [unwired: 2 in, 2 out]
                n185 = property on="Slider" class="Slide (strict)"("Visible"=FALSE) -> ()  [unwired: 2 in, 2 out]
              }
              frame Default {
                n186 = property on="Ring" class="Ring (strict)"("Visible"=FALSE) -> ()  [unwired: 2 in, 2 out]
                n187 = property on="Slider" class="Slide (strict)"("Visible"=FALSE) -> ()  [unwired: 2 in, 2 out]
              }
              frame "Brightness  **", "Color Level  **", "Compression  **", "FPS  **", "Sharpness  **" {
                n188 = call <vilib>:"NT Read Number.vi"("Name"=w315) -> ("Numeric"=w314:dbl)  [unwired: 9 in, 1 out]
                n189 = local write "Slider"(w314) -> ()
                n190 = property on="Slider" class="Slide (strict)"("Visible"=TRUE, "Scale.Maximum"=100.0 ("Scale.Range:Maximum")) -> ()  [unwired: 2 in, 2 out]
                n191 = property on="Ring" class="Ring (strict)"("Visible"=FALSE) -> ()  [unwired: 2 in, 2 out]
              }
            }
          }
        }
        n192 = property on="Progress" class="Clust (strict)"("Visible"=FALSE) -> ()  [unwired: 2 in, 2 out]
      }
      event "Test Name": Mouse Enter {
        # "Populate the ring with the list of tests"
        n193 = event-data() -> ()  [unwired: 1 in, 1 out]
        n194 = call <vilib>:"NT Read String Array.vi"("Name"="TestMode/TestList") -> ("String Array"=w322:string[])  [unwired: 9 in, 1 out]
        n195 = Build Array (concatenate)("Select the test to run...", w322) -> (w321:string[])
        n196 = property on="Test Name" class="Ring (strict)"("Strings []"=w321) -> ()  [unwired: 2 in, 2 out]
      }
      event "Test Name": Value Change {
        w324 = FALSE ("Visible")
        # "Tell the robot the test name to run"
        n197 = event-data() -> ("NewVal"=w328:u16)  [unwired: 1 in]
        n198 = property on="Test Name" class="Ring (strict)"() -> ("Strings []"=w329:string[])  [unwired: 2 in, 2 out]
        n199 = local write "Progress"(T5 {"Test Progress"=0, "Test Progress Text"=""} ("Progress")) -> ()
        n200 = Index Array(array=w329, index=w328) -> (element=w327:string)
        n201 = call <vilib>:"NT Write String.vi"("String"=w327, "Name"="TestMode/TestName") -> ()  [unwired: 9 in, 1 out]
        n202 = property on="Progress" class="Clust (strict)"("Visible"=TRUE) -> ()  [unwired: 2 in, 2 out]
        n203 = property on="Motor" class="Clust (strict)"("Visible"=w324) -> ()  [unwired: 2 in, 2 out]
        n204 = property on="Slider" class="Slide (strict)"("Visible"=w324) -> ()  [unwired: 2 in, 2 out]
        n205 = property on="On/Off" class="Bool (strict)"("Visible"=w324) -> ()  [unwired: 2 in, 2 out]
        n206 = property on="Rev/Fwd" class="Clust (strict)"("Visible"=w324) -> ()  [unwired: 2 in, 2 out]
        n207 = property on="Ring" class="Ring (strict)"("Visible"=w324) -> ()  [unwired: 2 in, 2 out]
      }
      event "Listbox": Double Click {
        n208 = event-data() -> ("PlatMods.Shift"=w332:bool, "Row"=w334:i32)  [unwired: 1 in]
        n209 = case shown="False" w332 {
          tunnel: w334 -> [w338 _]
          tunnel: 1 -> [w337 _]
          frame False {
            n210 = property on="Listbox" class="LstBox (strict)"() -> ("Item Symbols"=w336:i32[])  [unwired: 2 in, 2 out]
            n211 = Replace Array Subset(array=w336, new element=w337, index=w338) -> (w335:i32[])
            n212 = property on="Listbox" class="LstBox (strict)"("Item Symbols"=w335) -> ()  [unwired: 2 in, 2 out]
          }
          frame True {
            w339 = 0 ("Top Row")
            n213 = property on="Listbox" class="LstBox (strict)"() -> ("Number of Rows"=w341:u32)  [unwired: 2 in, 2 out]
            n214 = Initialize Array(0, w341) -> (w340:i32[])
            n215 = property on="Listbox" class="LstBox (strict)"("Top Row"=w339, "Value"=w339, "Item Symbols"=w340) -> ()  [unwired: 2 in, 2 out]
          }
        }
      }
      event "Listbox": Key Down {
        n216 = event-data() -> ("VKey"=w345:T10)  [unwired: 1 in]
        n217 = case shown="\"Left\", \"Right\"" w345 {
          selector: w345 -> [w350 _]
          tunnel: eventvkey."Left" ("VKey") -> [w348 _]
          frame "Left", "Right" {
            n218 = Equal?(x=w348, y=w350) -> (x = y?=w349:bool)
            n219 = Select(t=0, s=w349, f=1) -> (s? t:f=w351:i32)
            n220 = property on="Listbox" class="LstBox (strict)"() -> ("Item Symbols"=w354:i32[])  [unwired: 2 in, 2 out]
            n221 = Replace Array Subset(array=w354, new element=w351, index="Listbox") -> (w353:i32[])
            n222 = property on="Listbox" class="LstBox (strict)"("Item Symbols"=w353) -> ()  [unwired: 2 in, 2 out]
          }
          frame Default {
          }
        }
      }
      event "DB Camera Config": Value Change {
        n223 = event-data() -> ("NewVal"=w358:bool)  [unwired: 1 in]
        n224 = case shown="False" w358 {
          tunnel: w357 -> [w367 _]
          tunnel: [w360 w378] -> w356
          tunnel: w355 -> [w359 w378]
          frame False {
            w374 = "Camera"
            w377 = FALSE ("Visible")
            n225 = local read "Camera Settings"() -> (w366:T3)
            n226 = Index Array(array=w367) -> (element=w370:cluster{string[]})  [unwired: 1 in]
            n227 = Unbundle(w366) -> ("Frame Rate"=w365:i32, "Compression"=w364:i32, "Size"=w368:u16)
            n228 = Unbundle(w370) -> (w369:string[])
            n229 = Index Array(array=w369, index=w368) -> (element=w363:string)
            n230 = call-poly <vilib>:"Write Key.vi"("section"=w374, "value"=w363, "key"="Size", "refnum"=w359) -> ("refnum out"=w376:T9)  [unwired: 2 in, 5 out]
            n231 = call-poly <vilib>:"Write Key.vi"("section"=w374, "value"=w365, "key"="FrameRate", "refnum"=w376) -> ("refnum out"=w375:T9)  [unwired: 1 in, 6 out]
            n232 = property on="Camera Settings" class="Clust (strict)"("Visible"=w377) -> ()  [unwired: 2 in, 2 out]
            n233 = local write "DB Camera Config"(w377) -> ()
            n234 = call-poly <vilib>:"Write Key.vi"("section"=w374, "value"=w364, "key"="Compression", "refnum"=w375) -> ("refnum out"=w361:T9)  [unwired: 1 in, 6 out]
            n235 = call <vilib>:"Close Config Data.vi"("refnum"=w361) -> ("file path"=w362:path)  [unwired: 2 in, 8 out]
            n236 = call <vilib>:"Open Config Data.vi"("configuration file path"=w362) -> ("refnum"=w360:T9)  [unwired: 8 in, 2 out]
          }
          frame True {
            n237 = property on="Camera Settings" class="Clust (strict)"("Visible"=TRUE) -> ()  [unwired: 2 in, 2 out]
          }
        }
      }
      event "Camera Settings": Value Change {
        n238 = event-data() -> ("NewVal"=w391:T3)  [unwired: 1 in]
        n239 = Index Array(array=w387) -> (element=w386:cluster{string[]})  [unwired: 1 in]
        n240 = Unbundle(w391) -> ("Frame Rate"=w382:i32, "Compression"=w381:i32, "Size"=w384:u16)
        n241 = Unbundle(w386) -> (w385:string[])
        n242 = Index Array(array=w385, index=w384) -> (element=w383:string)
        n243 = Format Into String(format string="%s   %dfps   %d%%", w383, w382, w381) -> (resulting string=w388:string)  [unwired: 2 in, 1 out]
        n244 = Build Array(w388) -> (w389:string[])
        n245 = property on="DB Camera Config" class="Bool (strict)"("Strings [4]"=w389) -> ()  [unwired: 2 in, 2 out]
      }
      event "Motor.Enable": Value Change {
        n246 = event-data() -> ("NewVal"=w397:bool)  [unwired: 1 in]
        n247 = Unbundle("Motor") -> ("Value"=w396:dbl)  [unwired: 1 out]
        n248 = Select(t=w396, s=w397, f=0.0) -> (s? t:f=w394:dbl)
        n249 = call <vilib>:"NT Write Number.vi"("Numeric"=w394, "Name"=w393) -> ()  [unwired: 9 in, 1 out]
      }
      event "Slider": Value Change {
        n250 = event-data() -> ("NewVal"=w400:dbl)  [unwired: 1 in]
        n251 = call <vilib>:"NT Write Number.vi"("Numeric"=w400, "Name"=w401) -> ()  [unwired: 9 in, 1 out]
      }
      event "On/Off": Value Change {
        n252 = event-data() -> ("NewVal"=w405:bool)  [unwired: 1 in]
        n253 = Boolean To (0,1)(Boolean=w405) -> (0, 1=w404:i16)
        n254 = call <vilib>:"NT Write Number.vi"("Numeric"=w404, "Name"=w403) -> ()  [unwired: 9 in, 1 out]
      }
      event "Rev/Fwd": Value Change {
        n255 = event-data() -> ("NewVal.Forward"=w413:bool, "NewVal.Reverse"=w412:bool)  [unwired: 1 in]
        n256 = Boolean To (0,1)(Boolean=w413) -> (0, 1=w409:i16)
        n257 = Boolean To (0,1)(Boolean=w412) -> (0, 1=w411:i16)
        n258 = Negate(x=w411) -> (-x=w410:i16)
        n259 = Add(x=w409, y=w410) -> (x+y=w408:i16)
        n260 = call <vilib>:"NT Write Number.vi"("Numeric"=w408, "Name"=w407) -> ()  [unwired: 9 in, 1 out]
      }
      event "Ring": Value Change {
        n261 = event-data() -> ("NewVal"=w417:u16)  [unwired: 1 in]
        n262 = property on="Ring" class="Ring (strict)"() -> ("Strings []"=w418:string[])  [unwired: 2 in, 2 out]
        n263 = Index Array(array=w418, index=w417) -> (element=w416:string)
        n264 = call <vilib>:"NT Write String.vi"("String"=w416, "Name"=w415) -> ()  [unwired: 9 in, 1 out]
      }
    }
  }
  n265 = Index Array(array=w17) -> (element=w18:cluster{string[]})  [unwired: 1 in]
  n266 = Unbundle(w18) -> (w16:string[])
  n267 = Match First String(2:w16, 3:w15) -> (0:w14:i32)  [unwired: 1 out]
  n268 = Bundle("value"=w20, "value"=w19, "index"=w14) -> (w8:cluster{"value":i32, "value":i32, "index":i32})  [unwired: 1 out]
  n269 = property on="On/Off" class="Bool (strict)"("Visible"=w31) -> ()  [unwired: 2 in, 2 out]
  n270 = property on="Motor" class="Clust (strict)"("Visible"=w31) -> ()  [unwired: 2 in, 2 out]
  n271 = property on="Camera Settings" class="Clust (strict)"("Val(Sgnl)"=w8) -> ()  [unwired: 2 in, 2 out]
  n272 = property on="Rev/Fwd" class="Clust (strict)"("Visible"=w31) -> ()  [unwired: 2 in, 2 out]
  n273 = property on="Progress" class="Clust (strict)"("Visible"=w31) -> ()  [unwired: 2 in, 2 out]
  n274 = property on="Camera Settings" class="Clust (strict)"("Visible"=w31) -> ()  [unwired: 2 in, 2 out]
  n275 = local write "DB Camera Config"(w31) -> ()
  n276 = property on="Ring" class="Ring (strict)"("Visible"=w31) -> ()  [unwired: 2 in, 2 out]
